vi "analyseTemperature.vi"(8 "error in (no error)":errorcluster, 11 "TemperatureAnalyser in":refnum<class "TemperatureAnalyser.lvclass">) -> (0 "error out":errorcluster, 3 "TemperatureAnalyser out":refnum<class "TemperatureAnalyser.lvclass">)   [LabVIEW 2009, in "Tools.lvlib" / "Imaging.lvlib" / "TemperatureAnalyser.lvclass"]
uses:
  TemperatureAnalyser.lvclass
  Filing/FileSystem/FileSystem.lvclass
  ImageAnalyser.lvclass
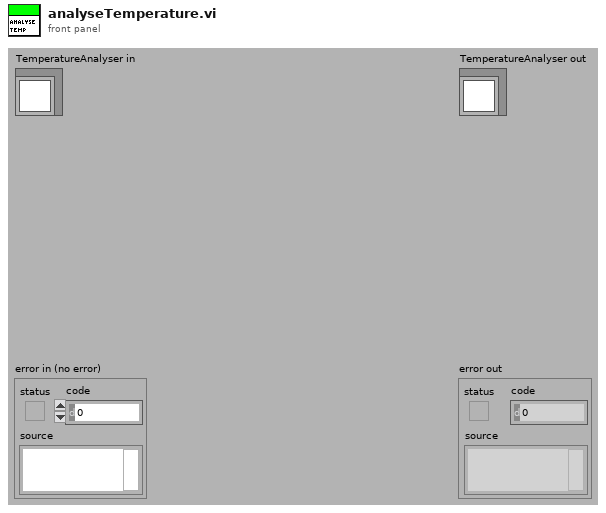
[diagram p1: front panel]
types:
  T1 = cluster{"Name":string, "Results":dbl[], "AnalysisType":string}
  T2 = cluster{"Name":string, "Results":dbl[], "AnalysisType":string}[]
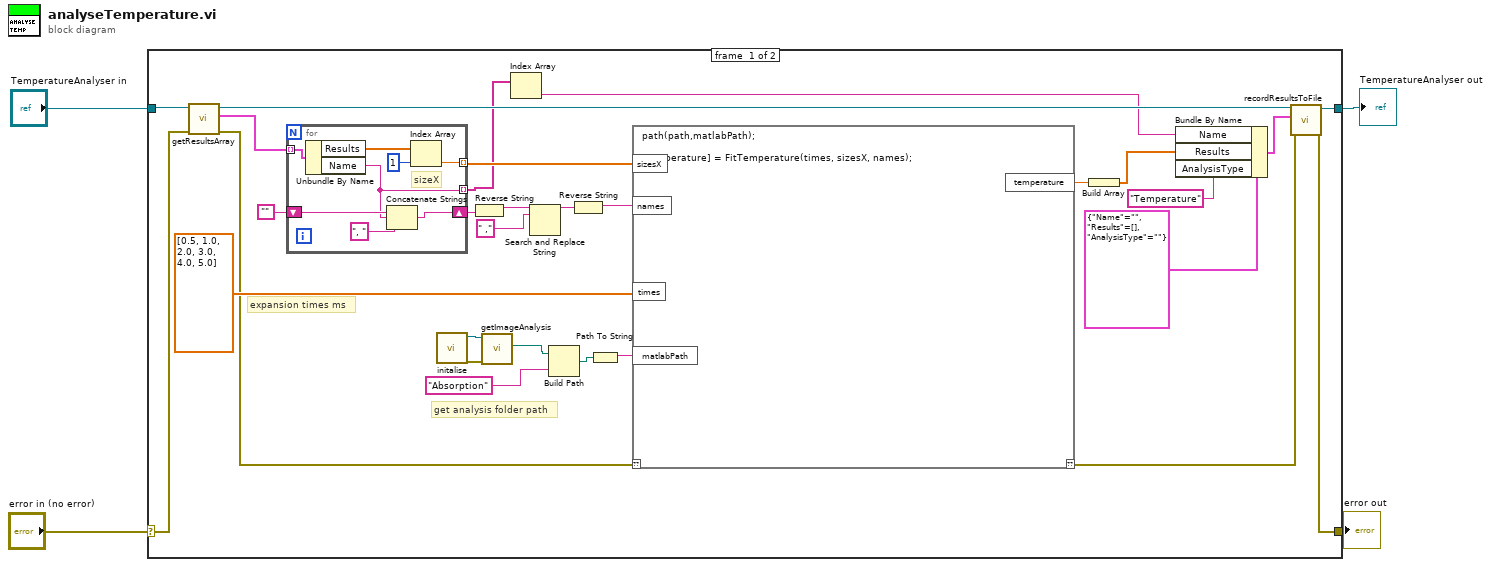
[diagram p0: block diagram]
diagram:
  n1 = case shown="No Error" "error in (no error)" {
    selector: "error in (no error)" -> [w17 w43]
    tunnel: [w5 w43] -> w3
    tunnel: [w15 w42] -> w1
    tunnel: "TemperatureAnalyser in" -> [w19 w42]
    frame #0 {
      # "get analysis folder path"
      # "expansion times ms"
      n2 = call "getResultsArray.vi"("error in (no error)"=w17, "ImageAnalyser in"=w19) -> ("error out"=w16:errorcluster, "resultsArray"=w18:T2, "ImageAnalyser out"=w14:refnum<class "TemperatureAnalyser.lvclass">)  [unwired: 7 in]
      n3 = for {
        tunnel: w18 -> [w41] mode=indexing
        tunnel: [w38] -> w33 mode=indexing
        shift-right: [w36] -> w30
        shift-left: "" -> [w35]
        tunnel: [w34] -> w8 mode=indexing
        # "sizeX"
        n4 = Unbundle By Name(w41) -> ("Results"=w40:dbl[], "Name"=w34:string)
        n5 = Concatenate Strings(w35, w34, ", ") -> (w36:string)
        n6 = Index Array(array=w40, index=1) -> (element=w38:dbl)
      }
      n7 = call "initalise.vi"() -> ("error out"=w25:errorcluster, "FileSystem out"=w26:refnum<class "FileSystem.lvclass">)  [unwired: 10 in]
      n8 = Reverse String(1:w30) -> (0:w29:string)
      n9 = call "getImageAnalysis.vi"("error in (no error)"=w25, "FileSystem in"=w26) -> ("ImageAnalysis"=w24:path)  [unwired: 7 in, 2 out]
      n10 = Index Array(array=w8) -> (element=w7:string)  [unwired: 1 in]
      n11 = Search and Replace String(input string=w29, search string=" ,") -> (result string=w27:string)  [unwired: 6 in, 3 out]
      n12 = Build Path(base path=w24, name or relative path="Absorption") -> (appended path=w22:path)
      n13 = Reverse String(1:w27) -> (0:w20:string)
      n14 = Path To String(path=w22) -> (string=w21:string)
      n15 = script code="path(path,matlabPath);\n\n[temperature] = FitTemperature(times, sizesX, names);"("??"=w16, "sizesX"=w33, "times"=dbl[] [0.5, 1.0, 2.0, 3.0, 4.0, 5.0], "matlabPath"=w21, "names"=w20) -> ("??"=w6:errorcluster, "temperature"=w13:dbl)
      n16 = Build Array(w13) -> (w10:dbl[])
      n17 = Bundle By Name(cluster=T1 {"Name"="", "Results"=[], "AnalysisType"=""} ("output cluster"), "Name"=w7, "Results"=w10, "AnalysisType"="Temperature") -> (w11:T1)
      n18 = call-dynamic "recordResultsToFile.vi"("error in (no error)"=w6, "Results"=w11, "ImageAnalyser in"=w14) -> ("error out"=w5:errorcluster, "ImageAnalyser out"=w15:refnum<class "TemperatureAnalyser.lvclass">)  [unwired: 7 in]
    }
    frame #1 {
    }
  }
  "error out" <- w3
  "TemperatureAnalyser out" <- w1
